vi "scope_init.vi"(0 "Vertical Coupling (1: DC)":i32(ring)=1 items=["AC", "DC", "Ground"], 1 "Vertical Range (10.0 V/div)":dbl=10.0, 6 "Timebase (0.0005 s)":dbl=0.0005, 8 "error in (no error)":errorcluster, 9 "Trigger Level (0.0 V)":dbl, 10 "Trigger Mode (0: Auto)":i32(ring) items=["Auto", "Normal"], 11 "VISA resource name":refnum<visa-resource-name>) -> (2 "error out":errorcluster, 3 "VISA resource name out":refnum<visa-resource-name>)   [LabVIEW 2015]
uses:
  <instrlib>/Tektronix TDS 200 1000 2000 Series/Public/Configure/Configure Trigger (Edge).vi
  <instrlib>/Tektronix TDS 200 1000 2000 Series/Tektronix TDS 200 1000 2000 Series.lvlib
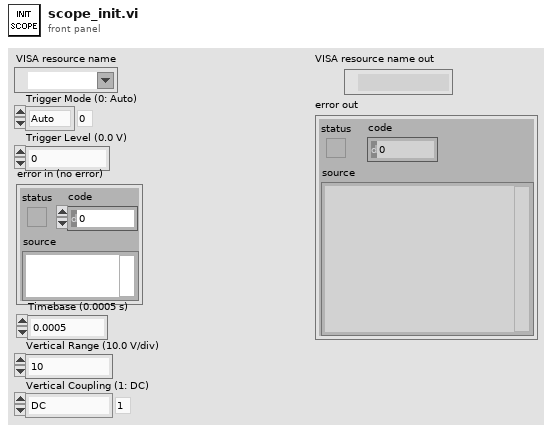
[diagram p1: front panel]
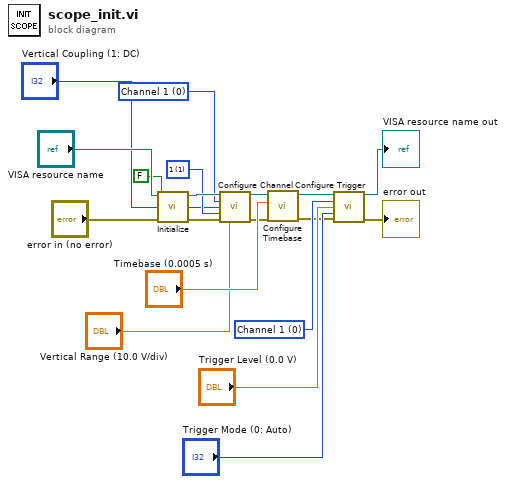
[diagram p0: block diagram]
diagram:
  w14 = 1 items=["1"=1, "10"=10, "20"=20, "50"=50, "100"=100, "500"=500, "1000"=1000] ("Probe Attenuation (10: 10X)")
  w15 = 0 items=["Channel 1", "Channel 2", "Channel 3", "Channel 4", "Math", "Reference A", "Reference B", "Reference C", "Reference D"] ("Channel (0: Channel 1)")
  w9 = 0 items=["Channel 1", "Channel 2", "Channel 3", "Channel 4", "External Input", "Attenuated External Input"] ("Trigger Source (0: Channel 1)")
  n1 = call <instrlib>:"Initialize.vi"("error in (no error)"="error in (no error)", "ID Query? (T: Yes)"=FALSE, "VISA resource name"="VISA resource name") -> ("error out"=w16:errorcluster, "VISA resource name out"=w17:refnum<visa-resource-name>)  [unwired: 7 in]
  n2 = call <instrlib>:"Configure Channel.vi"("VISA resource name"=w17, "Channel (0: Channel 1)"=w15, "Vertical Coupling (1: DC)"="Vertical Coupling (1: DC)", "Probe Attenuation (10: 10X)"=w14, "error in (no error)"=w16, "Vertical Range (10.0 V/div)"="Vertical Range (10.0 V/div)") -> ("VISA resource name out"=w10:refnum<visa-resource-name>, "error out"=w5:errorcluster)  [unwired: 8 in]
  n3 = call <instrlib>:"Configure Timebase.vi"("error in (no error)"=w5, "Timebase (0.0005 s)"="Timebase (0.0005 s)", "VISA resource name"=w10) -> ("error out"=w4:errorcluster, "VISA resource name out"=w11:refnum<visa-resource-name>)  [unwired: 7 in]
  n4 = call-poly <instrlib>:"Configure Trigger.vi"("VISA resource name"=w11, "Trigger Source (0: Channel 1)"=w9, "Trigger Level (0.0 V)"="Trigger Level (0.0 V)", "Trigger Mode (0: Auto)"="Trigger Mode (0: Auto)", "error in (no error)"=w4) -> ("VISA resource name out"=→"VISA resource name out":refnum<visa-resource-name>, "error out"=→"error out":errorcluster)  [unwired: 9 in]
